vi "Drive_Utils_getRobotState.vi"(8 "error in (no error)":errorcluster) -> (0 "error out":errorcluster, 3 "Robot State":T1)   [LabVIEW 2009, in "Drive.lvlib" / "Drive_Utils.lvlib"]
uses:
  Drive_Utils.lvlib
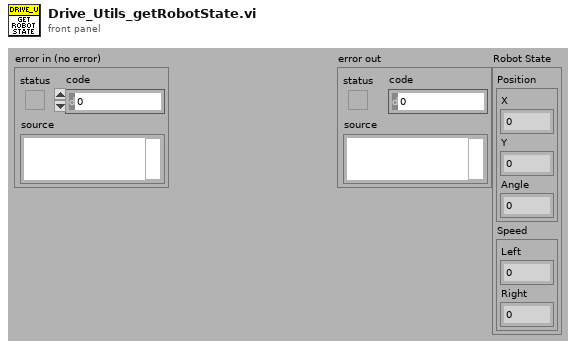
[diagram p1: front panel]
types:
  T1 = cluster{"Position":cluster{"X":dbl, "Y":dbl, "Angle":dbl}, "Speed":cluster{"Left":dbl, "Right":dbl}}
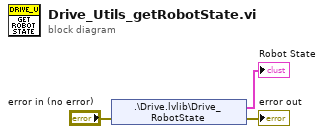
[diagram p0: block diagram]
diagram:
  n1 = shared-variable ".\\Drive.lvlib\\Drive_RobotState"(error in="error in (no error)") -> (→"Robot State":T1, error out=→"error out":errorcluster)
